vi "Main.vi"() -> ()   [LabVIEW 2013]
panel:
  out "rr":u32 format="%08x"
  out "ll":u32 format="%08x"
  out "Array":u64[](array[numeric]) format="%016x"
  out "L_Array":u32[](array[numeric]) format="%08x"
  out "R_Array":u32[](array[numeric]) format="%08x"
  out "Cipher":u64 format="%016x"
  in  "Key":u64=1086899994387671129 format="%016x"
  in  "Plain":u64=1316892562390803488 format="%016x"
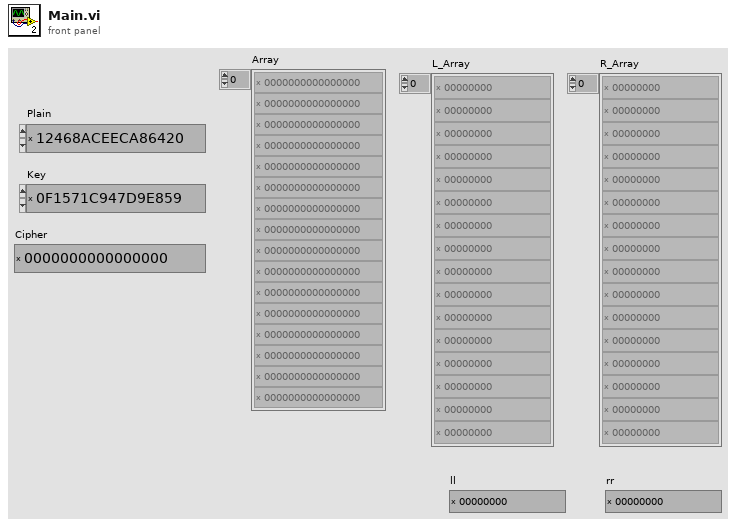
[diagram p1: front panel]
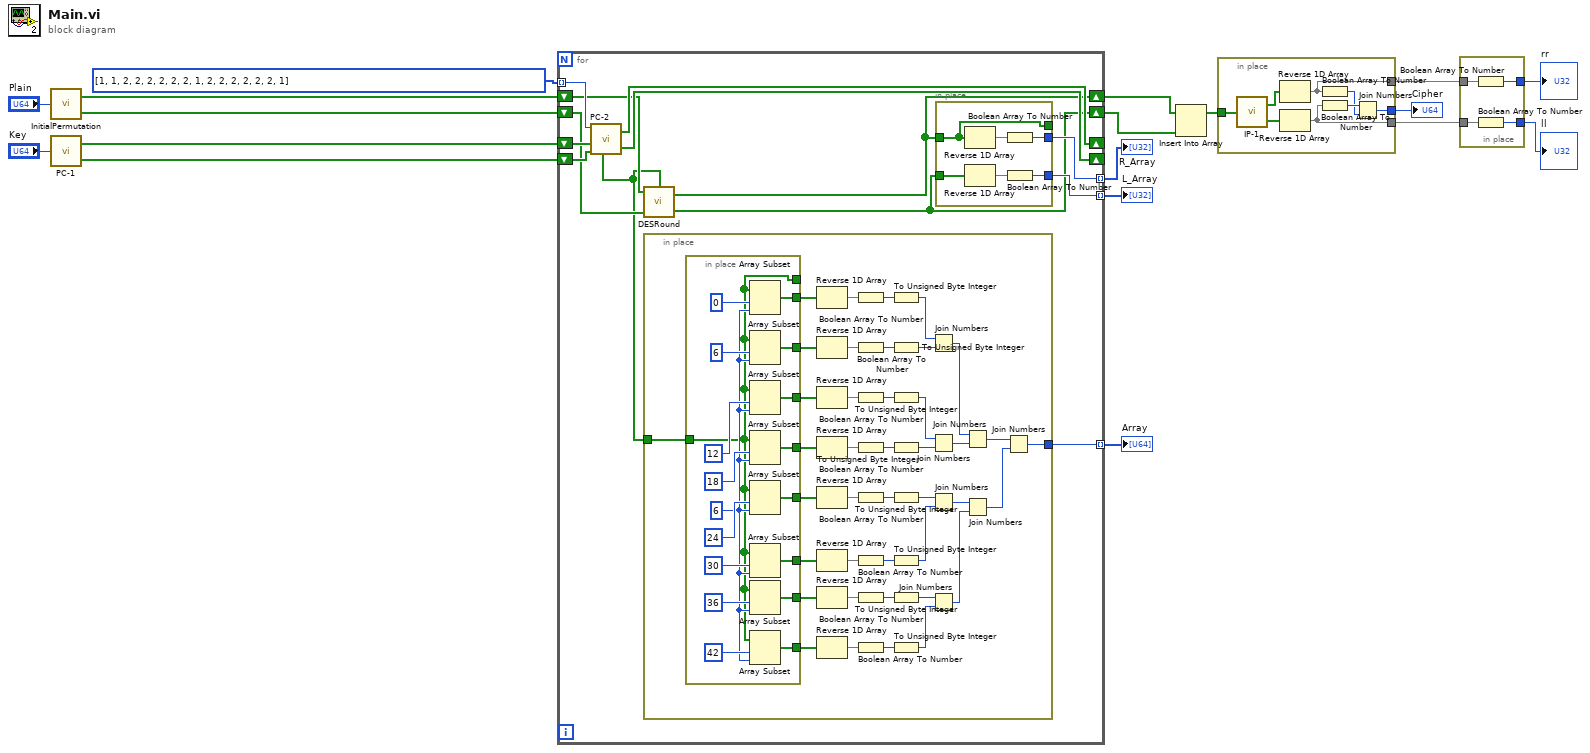
[diagram p0: block diagram]
diagram:
  n1 = call "InitialPermutation.vi"("Numeric"="Plain") -> ("Right"=w12:bool[], "Left"=w11:bool[])
  n2 = call "PC-1.vi"("Numeric"="Key") -> ("D"=w17:bool[], "C"=w16:bool[])
  n3 = for {
    shift-right: [w20] -> w1
    shift-left: w12 -> [w23]
    shift-right: [w19] -> w2
    shift-left: w11 -> [w24]
    shift-right: [w29] -> _
    shift-left: w17 -> [w31]
    shift-right: [w28] -> _
    shift-left: w16 -> [w30]
    tunnel: i32[] [1, 1, 2, 2, 2, 2, 2, 2, 1, 2, 2, 2, 2, 2, 2, 1] -> [w27] mode=indexing
    tunnel: [w26] -> w9 mode=indexing
    tunnel: [w25] -> w8 mode=indexing
    tunnel: [w21] -> w7 mode=indexing
    n4 = call "PC-2.vi"("Ci-1"=w30, "Di-1"=w31, "n"=w27) -> ("Ci"=w28:bool[], "Di"=w29:bool[], "SubKeyi"=w22:bool[])  [unwired: 2 in]
    n5 = call "DESRound.vi"("SubKey"=w22, "Left"=w24, "Right"=w23) -> ("NewLeft"=w19:bool[], "NewRight"=w20:bool[])  [unwired: 1 in]
    n6 = in-place {
      in-place-border: w22 -> [w71]
      in-place-border: [w40] -> w21
      n7 = in-place {
        in-place-border: [w72] -> _
        in-place-border: [w80] -> w70
        in-place-border: [w79] -> w65
        in-place-border: [w78] -> w62
        in-place-border: [w77] -> w59
        in-place-border: [w76] -> w56
        in-place-border: [w75] -> w49
        in-place-border: [w74] -> w48
        in-place-border: [w73] -> w47
        in-place-border: w71 -> [w72]
        w81 = 6 ("length")
        n8 = Array Subset(array=w72, index=0, length=w81) -> (w73:bool[])
        n9 = Array Subset(array=w72, index=6, length=w81) -> (w80:bool[])
        n10 = Array Subset(array=w72, index=12, length=w81) -> (w79:bool[])
        n11 = Array Subset(array=w72, index=18, length=w81) -> (w78:bool[])
        n12 = Array Subset(array=w72, index=24, length=w81) -> (w77:bool[])
        n13 = Array Subset(array=w72, index=30, length=w81) -> (w76:bool[])
        n14 = Array Subset(array=w72, index=36 ("length"), length=w81) -> (w75:bool[])
        n15 = Array Subset(array=w72, index=42, length=w81) -> (w74:bool[])
      }
      n16 = Reverse 1D Array(array=w47) -> (reversed array=w50:bool[])
      n17 = Reverse 1D Array(array=w70) -> (reversed array=w69:bool[])
      n18 = Reverse 1D Array(array=w65) -> (reversed array=w66:bool[])
      n19 = Reverse 1D Array(array=w62) -> (reversed array=w64:bool[])
      n20 = Reverse 1D Array(array=w59) -> (reversed array=w60:bool[])
      n21 = Reverse 1D Array(array=w56) -> (reversed array=w58:bool[])
      n22 = Reverse 1D Array(array=w49) -> (reversed array=w54:bool[])
      n23 = Reverse 1D Array(array=w48) -> (reversed array=w53:bool[])
      n24 = Boolean Array To Number(Boolean array=w50) -> (number=w51:u32)
      n25 = Boolean Array To Number(Boolean array=w69) -> (number=w68:u32)
      n26 = Boolean Array To Number(Boolean array=w66) -> (number=w67:u32)
      n27 = Boolean Array To Number(Boolean array=w64) -> (number=w63:u32)
      n28 = Boolean Array To Number(Boolean array=w60) -> (number=w61:u32)
      n29 = Boolean Array To Number(Boolean array=w58) -> (number=w57:u32)
      n30 = Boolean Array To Number(Boolean array=w54) -> (number=w55:u32)
      n31 = Boolean Array To Number(Boolean array=w53) -> (number=w52:u32)
      n32 = To Unsigned Byte Integer(number=w51) -> (unsigned 8bit integer=w39:u8)
      n33 = To Unsigned Byte Integer(number=w68) -> (unsigned 8bit integer=w38:u8)
      n34 = To Unsigned Byte Integer(number=w67) -> (unsigned 8bit integer=w35:u8)
      n35 = To Unsigned Byte Integer(number=w63) -> (unsigned 8bit integer=w34:u8)
      n36 = To Unsigned Byte Integer(number=w61) -> (unsigned 8bit integer=w32:u8)
      n37 = To Unsigned Byte Integer(number=w57) -> (unsigned 8bit integer=w33:u8)
      n38 = To Unsigned Byte Integer(number=w55) -> (unsigned 8bit integer=w36:u8)
      n39 = To Unsigned Byte Integer(number=w52) -> (unsigned 8bit integer=w37:u8)
      n40 = Join Numbers(hi=w39, lo=w38) -> ((hi.lo)=w46:u16)
      n41 = Join Numbers(hi=w35, lo=w34) -> ((hi.lo)=w45:u16)
      n42 = Join Numbers(hi=w32, lo=w33) -> ((hi.lo)=w44:u16)
      n43 = Join Numbers(hi=w36, lo=w37) -> ((hi.lo)=w43:u16)
      n44 = Join Numbers(hi=w46, lo=w45) -> ((hi.lo)=w42:u32)
      n45 = Join Numbers(hi=w44, lo=w43) -> ((hi.lo)=w41:u32)
      n46 = Join Numbers(hi=w42, lo=w41) -> ((hi.lo)=w40:u64)
    }
    n47 = in-place {
      in-place-border: [w94] -> w26
      in-place-border: [w93] -> w25
      in-place-border: w19 -> [w91]
      in-place-border: [w90] -> _
      in-place-border: w20 -> [w90]
      n48 = Reverse 1D Array(array=w90) -> (reversed array=w95:bool[])
      n49 = Reverse 1D Array(array=w91) -> (reversed array=w92:bool[])
      n50 = Boolean Array To Number(Boolean array=w95) -> (number=w94:u32)
      n51 = Boolean Array To Number(Boolean array=w92) -> (number=w93:u32)
    }
  }
  "R_Array" <- w9
  "L_Array" <- w8
  "Array" <- w7
  n52 = Insert Into Array(array=w1, new element=w2) -> (w10:bool[])  [unwired: 1 in]
  n53 = in-place {
    in-place-border: [w101] -> w15
    in-place-border: w10 -> [w98]
    in-place-border: [w97] -> w6
    in-place-border: [w96] -> w5
    n54 = call "IP-1.vi"("array"=w98) -> ("Right"=w100:bool[], "Left"=w99:bool[])
    n55 = Reverse 1D Array(array=w100) -> (reversed array=w96:bool[])
    n56 = Reverse 1D Array(array=w99) -> (reversed array=w97:bool[])
    n57 = Boolean Array To Number(Boolean array=w96) -> (number=w102:u32)
    n58 = Boolean Array To Number(Boolean array=w97) -> (number=w103:u32)
    n59 = Join Numbers(hi=w103, lo=w102) -> ((hi.lo)=w101:u64)
  }
  "Cipher" <- w15
  n60 = in-place {
    in-place-border: [w107] -> w4
    in-place-border: [w106] -> w3
    in-place-border: w5 -> [w104]
    in-place-border: w6 -> [w105]
    n61 = Boolean Array To Number(Boolean array=w104) -> (number=w106:u32)
    n62 = Boolean Array To Number(Boolean array=w105) -> (number=w107:u32)
  }
  "ll" <- w4
  "rr" <- w3
